vi "Main.vi"(11 "Module Admin":refnum<class "Delacor_lib_QMH_Cloneable Module Admin.lvclass">) -> ()   [LabVIEW 2024, in "Cloneable Subpanel.lvlib"]
doc: "This template is based off of the Queued Message Handler design pattern and the Queued Message Handler project template that ships with LabVIEW.\n\nThe main difference is that the queue is private to this module and communication between modules is performed via Broadcast and Request events.\n\nRequest events are wrapped in public API methods and are handled in the Event Handling Loop (EHL) of this VI. Any module can register for Broadcast events sent by this module. The EHL generates messages based on user interface actions.\n\nThe Message Handling Loop (MHL) processes messages generated by the EHL, or by other messages. The messages are string values, so new messages can be added easily to the Message Cases case structure in the MHL. Each message cluster can also provide an optional value for Message Data, which is a variant that can be converted to whatever message-specific data is required.\n_____\nBased on DQMH Dev Tools: Project Template 7.1.0.1499."
uses:
  Cloneable Subpanel.lvlib
  <vilib>/Delacor/Delacor QMH/Libraries/Message Queue_class/Delacor_lib_QMH_Message Queue.lvclass
  Module Data--cluster.ctl
  <vilib>/Utility/miscctls.llb/LVPointTypeDef.ctl
  <vilib>/Delacor/Delacor QMH/Libraries/Message Queue_class/Delacor_lib_QMH_Enqueue Message (Single).vi
  Stop Argument--cluster.ctl
  <vilib>/Delacor/Delacor QMH/Libraries/Cloneable Module Admin_class/Delacor_lib_QMH_Cloneable Module Admin.lvclass
  Draw FP in SubPanel Argument--cluster.ctl
  Remove from SubPanel Argument--cluster.ctl
panel:
  out "error out":errorcluster
  out "Status":string
  in  "Simulate EHL Error":bool
  in  "Simulate MHL Error":bool
  # "Other processes communicate with this Module via its Public API (wrappers for its Request Events).\n\nThis Module communicates with other processes via its Broadcast Events.\nAny process that wants to receive these messages can register for this module's Broadcast events."
  # "This template is for the DQMH framework. See the block diagram for more information on how to use this template."
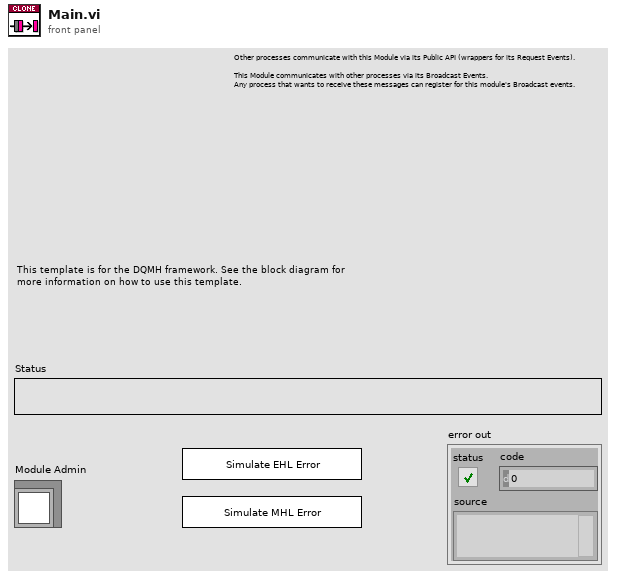
[diagram p1: front panel]
types:
  T1 = typedef "Cloneable Subpanel.lvlib/Request Events--cluster.ctl" = cluster{"Stop Module":refnum<user-event>, "Show Panel":refnum<user-event>, "Hide Panel":refnum<user-event>, "Show Diagram":refnum<user-event>, "Get Module Execution Status":refnum<user-event>, "Draw FP in SubPanel":refnum<user-event>, "Remove from SubPanel":refnum<user-event>}
  T2 = typedef "Cloneable Subpanel.lvlib/Module Data--cluster.ctl" = cluster{"Status":string, "Sub Panel":refnum<vi>}
  T3 = enum32{"invalid lock state", "Not Locked", "Locked (No Password)", "Password-protected"}
  T4 = typedef "Cloneable Subpanel.lvlib/Stop Argument--cluster.ctl" = cluster{"Module ID":i32, "Origin":string, "Exit via Stop Module Req?":bool, "Wait for Module to stop?":bool}
  T5 = typedef "Cloneable Subpanel.lvlib/Draw FP in SubPanel Argument--cluster.ctl" = cluster{"Module ID":i32, "Sub Panel":refnum<vi>}
  T6 = typedef "Cloneable Subpanel.lvlib/Remove from SubPanel Argument--cluster.ctl" = cluster{"Module ID":i32, "Boolean":bool}
  T7 = typedef "LVPointTypeDef.ctl" = cluster{"Horizontal":i16, "Vertical":i16}
  T8 = enum32{"Invalid", "Standard", "Closed", "Hidden", "Minimized", "Maximized"}
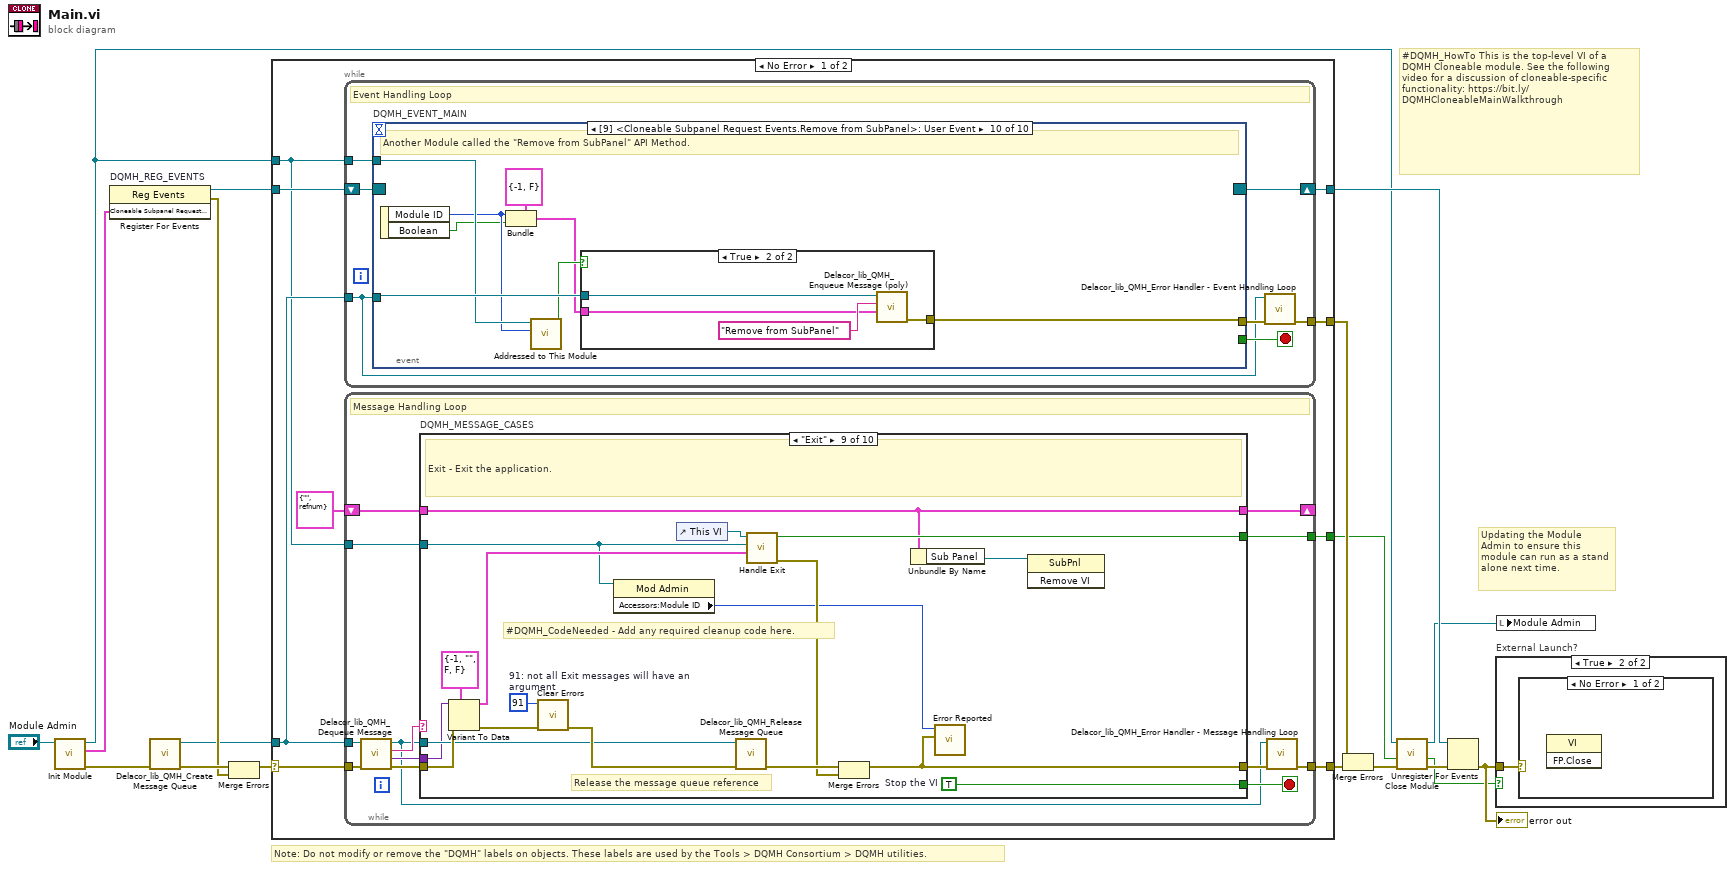
[diagram p0: block diagram]
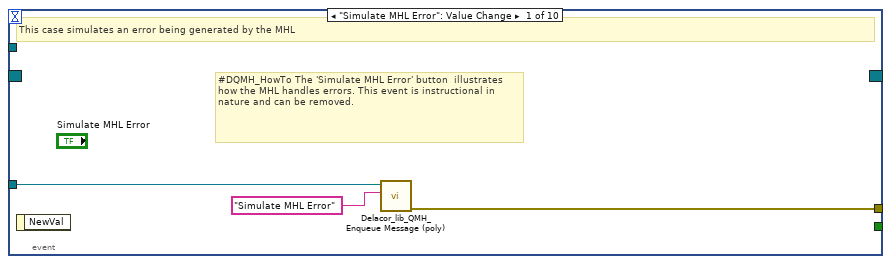
[diagram p2: hidden frame]
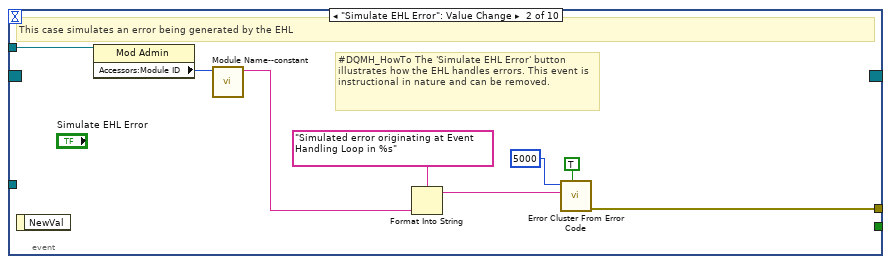
[diagram p3: hidden frame]
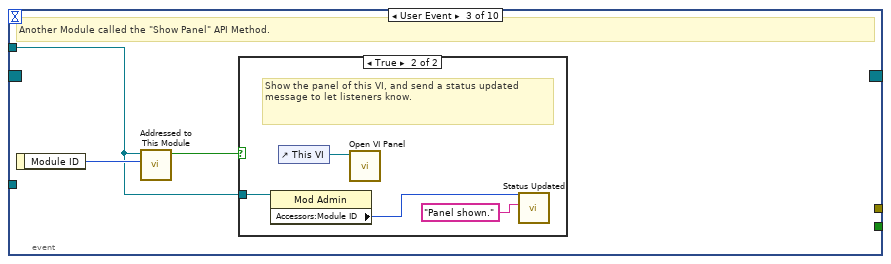
[diagram p4: hidden frame]
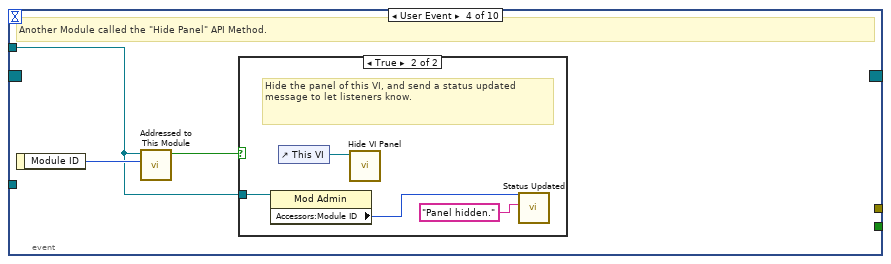
[diagram p6: hidden frame]
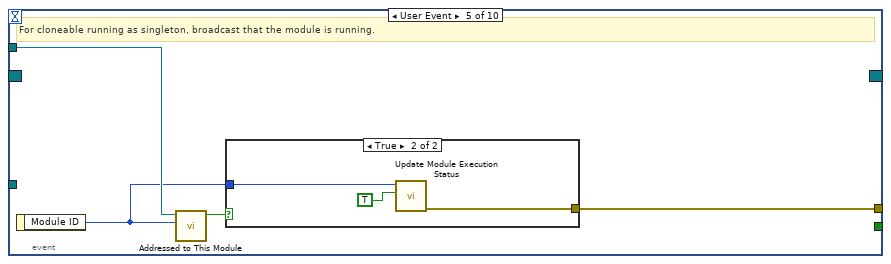
[diagram p8: hidden frame]
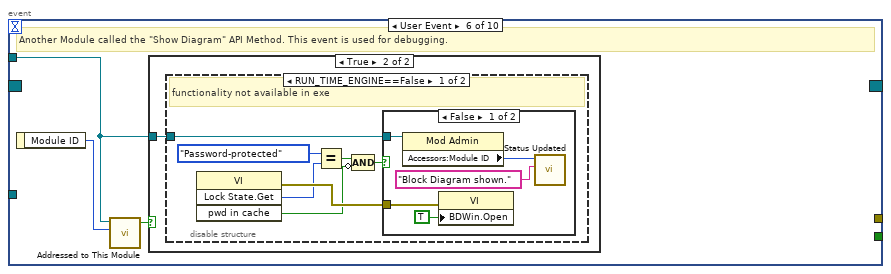
[diagram p10: hidden frame]
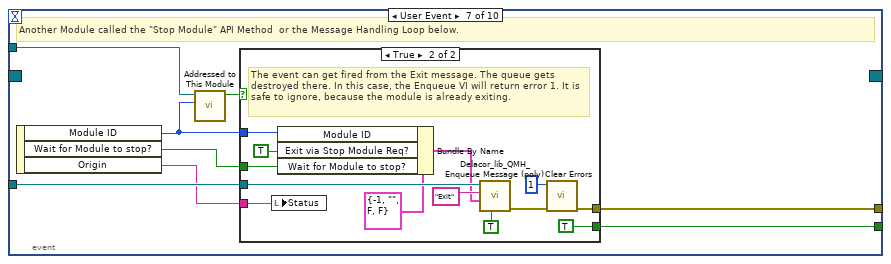
[diagram p14: hidden frame]
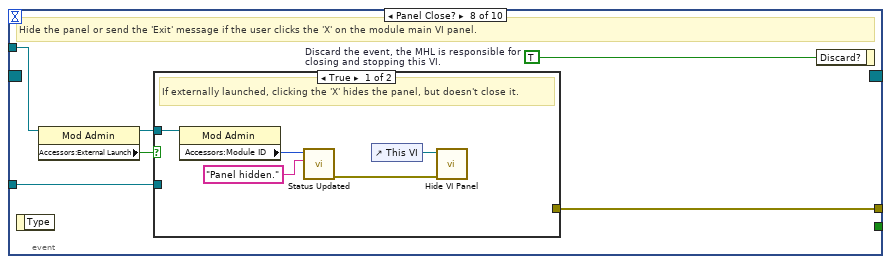
[diagram p16: hidden frame]
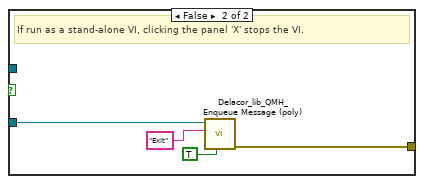
[diagram p17: hidden frame]
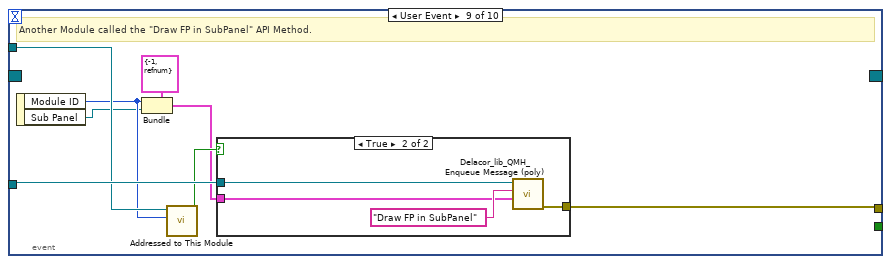
[diagram p18: hidden frame]
diagram:
  # "#DQMH_HowTo This is the top-level VI of a DQMH Cloneable module. See the following video for a discussion of cloneable-specific functionality: https://bit.ly/DQMHCloneableMainWalkthrough"
  # "Note: Do not modify or remove the \"DQMH\" labels on objects. These labels are used by the Tools > DQMH Consortium > DQMH utilities."
  # "Updating the Module Admin to ensure this module can run as a stand alone next time."
  n1 = call "Init Module.vi"("Cloneable Module Admin in"="Module Admin") -> ("error out"=w15:errorcluster, "Cloneable Subpanel Request Events"=w7:T1, "Cloneable Module Admin out"=w4:refnum<class "Delacor_lib_QMH_Cloneable Module Admin.lvclass">)  [unwired: 8 in]
  n2 = register-events "DQMH_REG_EVENTS"(w7) -> (reference out=w8:refnum<event-registration>, error out=w10:errorcluster)  [unwired: 2 in]
  n3 = call <vilib>:"Delacor_lib_QMH_Create Message Queue.vi"("error in"=w15) -> ("error out"=w12:errorcluster, "Message Queue"=w6:refnum<class "Delacor_lib_QMH_Message Queue.lvclass">)  [unwired: 9 in]
  n4 = Merge Errors(w12, w10) -> (w11:errorcluster)
  n5 = case shown="No Error" w11 {
    selector: w11 -> [w25 w287]
    tunnel: [w27 w286] -> w16
    tunnel: [w24 w285] -> w9
    tunnel: w8 -> [w22 w285]
    tunnel: w6 -> [w21 w278]
    tunnel: [w26 _] -> w17
    tunnel: w4 -> [w20 w281]
    tunnel: [w19 _] -> w2
    frame No Error {
      n6 = while {
        tunnel: w21 -> [w28]
        shift-right: [w31] -> w24
        shift-left: w22 -> [w32]
        tunnel: [w33] -> w26
        tunnel: w20 -> [w29]
        stop <- w30 stop-if-true
        # "Event Handling Loop"
        n7 = event "DQMH_EVENT_MAIN" shown="[9] <Cloneable Subpanel Request Events.Remove from SubPanel>: User Event" {
          selector: w32 -> [_ _ _ _ _ _ _ _ _ _]
          dyn-events: [_ _ _ _ _ _ _ _ _ _] -> w31
          timeout: _ -> [_ _ _ _ _ _ _ _ _ _]
          tunnel: [_ _ _ _ _ _ w86 _ _ _] -> w30
          tunnel: w28 -> [w36 _ _ _ _ _ w89 w106 w126 w138]
          tunnel: [w37 w45 _ _ w63 _ w90 w109 w119 w131] -> w34
          tunnel: w29 -> [_ w44 w46 w53 w61 w67 w88 w107 w124 w136]
          event "Simulate MHL Error": Value Change {
            # "#DQMH_HowTo The 'Simulate MHL Error' button  illustrates how the MHL handles errors. This event is instructional in nature and can be removed."
            # "This case simulates an error being generated by the MHL"
            n8 = event-data() -> ()  [unwired: 1 in, 1 out]
            n9 = call-poly <vilib>:"Delacor_lib_QMH_Enqueue Message (poly).vi"("Message"="Simulate MHL Error", "Message Queue in"=w36) -> ("error out"=w37:errorcluster)  [unwired: 8 in, 1 out]
          }
          event "Simulate EHL Error": Value Change {
            # "#DQMH_HowTo The 'Simulate EHL Error' button  illustrates how the EHL handles errors. This event is instructional in nature and can be removed."
            # "This case simulates an error being generated by the EHL"
            n10 = event-data() -> ()  [unwired: 1 in, 1 out]
            n11 = property on="Property Node" class="Mod Admin"(reference=w44) -> ("Accessors:Module ID"=w43:i32)  [unwired: 1 in, 2 out]
            n12 = call "Module Name--constant.vi"("Module ID"=w43) -> ("Module Name"=w38:string)  [unwired: 10 in]
            n13 = Format Into String(format string="Simulated error originating at Event Handling Loop in %s", w38) -> (resulting string=w41:string)  [unwired: 2 in, 1 out]
            n14 = call <vilib>:"Error Cluster From Error Code.vi"("show call chain? (False)"=TRUE, "error message (\"\")"=w41, "error code (0)"=5000) -> ("error out"=w45:errorcluster)  [unwired: 6 in]
          }
          event User Event {
            # "Another Module called the \"Show Panel\" API Method."
            n15 = event-data() -> ("Module ID"=w47:i32)  [unwired: 1 in]
            n16 = call "Addressed to This Module.vi"("Module ID from Argument"=w47, "Module Admin"=w46) -> ("Addressed to this instance?"=w48:bool)  [unwired: 8 in, 1 out]
            n17 = case shown="True" w48 {
              tunnel: w46 -> [_ w50]
              frame False {
              }
              frame True {
                # "Show the panel of this VI, and send a status updated message to let listeners know."
                n18 = property on="Property Node" class="Mod Admin"(reference=w50) -> ("Accessors:Module ID"=w49:i32)  [unwired: 1 in, 2 out]
                n19 = control-ref of="This VI"() -> (w52:refnum<vi>)
                n20 = call "Open VI Panel.vi"("VI"=w52) -> ()  [unwired: 10 in, 1 out]
                n21 = call "Status Updated.vi"("Status"="Panel shown." ("format string"), "Module ID"=w49) -> ()  [unwired: 9 in, 1 out]
              }
            }
          }
          event User Event {
            # "Another Module called the \"Hide Panel\" API Method."
            n22 = event-data() -> ("Module ID"=w54:i32)  [unwired: 1 in]
            n23 = call "Addressed to This Module.vi"("Module ID from Argument"=w54, "Module Admin"=w53) -> ("Addressed to this instance?"=w55:bool)  [unwired: 8 in, 1 out]
            n24 = case shown="True" w55 {
              tunnel: w53 -> [_ w57]
              frame False {
              }
              frame True {
                # "Hide the panel of this VI, and send a status updated message to let listeners know."
                n25 = property on="Property Node" class="Mod Admin"(reference=w57) -> ("Accessors:Module ID"=w56:i32)  [unwired: 1 in, 2 out]
                n26 = control-ref of="This VI"() -> (w59:refnum<vi>)
                n27 = call "Hide VI Panel.vi"("VI"=w59) -> ()  [unwired: 10 in, 1 out]
                n28 = call "Status Updated.vi"("Status"="Panel hidden." ("format string"), "Module ID"=w56) -> ()  [unwired: 9 in, 1 out]
              }
            }
          }
          event User Event {
            # "For cloneable running as singleton, broadcast that the module is running."
            n29 = event-data() -> ("Module ID"=w60:i32)  [unwired: 1 in]
            n30 = call "Addressed to This Module.vi"("Module ID from Argument"=w60, "Module Admin"=w61) -> ("Addressed to this instance?"=w62:bool)  [unwired: 8 in, 1 out]
            n31 = case shown="True" w62 {
              tunnel: [_ w66] -> w63
              tunnel: w60 -> [_ w65]
              frame False {
              }
              frame True {
                n32 = call "Update Module Execution Status.vi"("Running?"=TRUE, "Module ID"=w65) -> ("error out"=w66:errorcluster)  [unwired: 9 in]
              }
            }
          }
          event User Event {
            # "Another Module called the \"Show Diagram\" API Method. This event is used for debugging."
            n33 = event-data() -> ("Module ID"=w68:i32)  [unwired: 1 in]
            n34 = call "Addressed to This Module.vi"("Module ID from Argument"=w68, "Module Admin"=w67) -> ("Addressed to this instance?"=w69:bool)  [unwired: 8 in, 1 out]
            n35 = case shown="True" w69 {
              tunnel: w67 -> [_ w70]
              frame False {
              }
              frame True {
                n36 = disable-structure shown="RUN_TIME_ENGINE==False" {
                  disable-tunnel: w70 -> [w71 _]
                  frame condition #0 (active) {
                    # "functionality not available in exe"
                    n37 = invoke on="Invoke Node" class="VI" method="Lock State.Get"() -> (error out=w77:errorcluster, "Get Lock State"=w76:T3, "pwd in cache"=w73:bool)  [unwired: 4 in, 1 out]
                    n38 = Equal?(x=T3."Password-protected", y=w76) -> (x = y?=w74:bool)
                    n39 = Compound Arithmetic op=AND(w74, invert w73) -> (w72:bool)
                    n40 = case shown="False" w72 {
                      tunnel: w77 -> [w82 _]
                      tunnel: w71 -> [w79 _]
                      frame False {
                        n41 = property on="Property Node" class="Mod Admin"(reference=w79) -> ("Accessors:Module ID"=w78:i32)  [unwired: 1 in, 2 out]
                        n42 = property on="Property Node" class="VI"(error in=w82, "BDWin.Open"=TRUE ("Block Diagram Window:Open")) -> ()  [unwired: 1 in, 2 out]
                        n43 = call "Status Updated.vi"("Status"="Block Diagram shown." ("format string"), "Module ID"=w78) -> ()  [unwired: 9 in, 1 out]
                      }
                      frame True {
                        # "Password-protected VI, and the password is not in the cache. Do not show the diagram."
                      }
                    }
                  }
                  frame condition #1 {
                  }
                }
              }
            }
          }
          event User Event {
            # "Another Module called the \"Stop Module\" API Method  or the Message Handling Loop below."
            n44 = event-data() -> ("Module ID"=w84:i32, "Wait for Module to stop?"=w85:bool, "Origin"=w83:string)  [unwired: 1 in]
            n45 = call "Addressed to This Module.vi"("Module ID from Argument"=w84, "Module Admin"=w88) -> ("Addressed to this instance?"=w87:bool)  [unwired: 8 in, 1 out]
            n46 = case shown="True" w87 {
              tunnel: [_ w102] -> w90
              tunnel: w89 -> [_ w98]
              tunnel: [_ TRUE] -> w86
              tunnel: w85 -> [_ w93]
              tunnel: w84 -> [_ w95]
              tunnel: w83 -> [_ w91]
              frame False {
              }
              frame True {
                # "The event can get fired from the Exit message. The queue gets destroyed there. In this case, the Enqueue VI will return error 1. It is safe to ignore, because the module is already exiting."
                n47 = local write "Status"(w91) -> ()
                n48 = Bundle By Name(cluster=T4 {"Module ID"=-1, "Origin"="", "Exit via Stop Module Req?"=FALSE, "Wait for Module to stop?"=FALSE} ("Stop Argument"), "Module ID"=w95, "Exit via Stop Module Req?"=TRUE, "Wait for Module to stop?"=w93) -> (w92:T4)
                n49 = call-poly <vilib>:"Delacor_lib_QMH_Enqueue Message (poly).vi"("Priority Message? (F)"=TRUE, "Message Data"=w92, "Message"="Exit", "Message Queue in"=w98) -> ("error out"=w103:errorcluster)  [unwired: 6 in, 1 out]
                n50 = call <vilib>:"Clear Errors.vi"("error in (no error)"=w103, "specific error code to clear (0: all)"=1) -> ("error out"=w102:errorcluster)  [unwired: 4 in, 1 out]
              }
            }
          }
          event Panel Close? {
            w108 = TRUE  # Discard the event, the MHL is responsible for closing and stopping this VI.
            # "Hide the panel or send the 'Exit' message if the user clicks the 'X' on the module main VI panel."
            n51 = event-data() -> ()  [unwired: 1 in, 1 out]
            n52 = property on="Property Node" class="Mod Admin"(reference=w107) -> (reference out=w104:refnum<class "Delacor_lib_QMH_Cloneable Module Admin.lvclass">, "Accessors:External Launch"=w105:bool)  [unwired: 1 in, 1 out]
            n53 = case shown="True" w105 {
              tunnel: w106 -> [_ w117]
              tunnel: [_ w118] -> w109
              tunnel: w104 -> [w112 _]
              frame True {
                # "If externally launched, clicking the 'X' hides the panel, but doesn't close it."
                n54 = property on="Property Node" class="Mod Admin"(reference=w112) -> ("Accessors:Module ID"=w111:i32)  [unwired: 1 in, 2 out]
                n55 = call "Status Updated.vi"("Status"="Panel hidden." ("format string"), "Module ID"=w111) -> ("error out"=w110:errorcluster)  [unwired: 9 in]
                n56 = control-ref of="This VI"() -> (w114:refnum<vi>)
                n57 = call "Hide VI Panel.vi"("error in"=w110, "VI"=w114) -> ()  [unwired: 9 in, 1 out]
              }
              frame False {
                # "If run as a stand-alone VI, clicking the panel 'X' stops the VI."
                n58 = call-poly <vilib>:"Delacor_lib_QMH_Enqueue Message (poly).vi"("Priority Message? (F)"=TRUE, "Message"="Exit", "Message Queue in"=w117) -> ("error out"=w118:errorcluster)  [unwired: 7 in, 1 out]
              }
            }
            n59 = event-data ("Event Filter Node")("Discard?"=w108) -> ()  [unwired: 1 in, 1 out]
          }
          event User Event {
            # "Another Module called the \"Draw FP in SubPanel\" API Method."
            n60 = event-data() -> ("Module ID"=w121:i32, "Sub Panel"=w120:refnum<vi>)  [unwired: 1 in]
            n61 = Bundle(cluster=T5 {"Module ID"=-1, "Sub Panel"=refnum} ("Draw FP in SubPanel Argument"), "Module ID"=w121, "Sub Panel"=w120) -> (w122:T5)
            n62 = call "Addressed to This Module.vi"("Module ID from Argument"=w121, "Module Admin"=w124) -> ("Addressed to this instance?"=w125:bool)  [unwired: 8 in, 1 out]
            n63 = case shown="True" w125 {
              tunnel: w126 -> [_ w130]
              tunnel: w122 -> [_ w128]
              tunnel: [_ w127] -> w119
              frame False {
              }
              frame True {
                n64 = call-poly <vilib>:"Delacor_lib_QMH_Enqueue Message (poly).vi"("Message Data"=w128, "Message"="Draw FP in SubPanel", "Message Queue in"=w130) -> ("error out"=w127:errorcluster)  [unwired: 7 in, 1 out]
              }
            }
          }
          event User Event {
            # "Another Module called the \"Remove from SubPanel\" API Method."
            n65 = event-data() -> ("Module ID"=w133:i32, "Boolean"=w132:bool)  [unwired: 1 in]
            n66 = Bundle(cluster=T6 {"Module ID"=-1, "Boolean"=FALSE} ("Remove from SubPanel Argument"), "Module ID"=w133, "Boolean"=w132) -> (w134:T6)
            n67 = call "Addressed to This Module.vi"("Module ID from Argument"=w133, "Module Admin"=w136) -> ("Addressed to this instance?"=w137:bool)  [unwired: 8 in, 1 out]
            n68 = case shown="True" w137 {
              tunnel: w138 -> [_ w142]
              tunnel: w134 -> [_ w140]
              tunnel: [_ w139] -> w131
              frame False {
              }
              frame True {
                n69 = call-poly <vilib>:"Delacor_lib_QMH_Enqueue Message (poly).vi"("Message Data"=w140, "Message"="Remove from SubPanel", "Message Queue in"=w142) -> ("error out"=w139:errorcluster)  [unwired: 7 in, 1 out]
              }
            }
          }
        }
        n70 = call-dynamic "Delacor_lib_QMH_Error Handler - Event Handling Loop.vi"("error in"=w34, "Message Queue in"=w28) -> ("dup error in"=w33:errorcluster)  [unwired: 8 in, 1 out]
      }
      n71 = while {
        tunnel: w21 -> [w143]
        shift-right: [w150] -> _
        shift-left: T2 {"Status"="", "Sub Panel"=refnum} ("Data Cluster") -> [w151]
        tunnel: w25 -> [w154]
        tunnel: [w152] -> w27
        tunnel: w20 -> [w145]
        tunnel: [w144] -> w19
        stop <- w149 stop-if-true
        # "Message Handling Loop"
        n72 = call-dynamic "Delacor_lib_QMH_Dequeue Message.vi"("error in"=w154, "Message Queue in"=w143) -> ("error out"=w153:errorcluster, "Message Data"=w147:variant, "Message"=w148:string, "Message Queue out"=w146:refnum<class "Delacor_lib_QMH_Message Queue.lvclass">)  [unwired: 6 in]
        n73 = case "DQMH_MESSAGE_CASES" shown="\"Exit\"" w148 {
          selector: w148 -> [_ _ _ _ _ _ _ _ _ w267]
          tunnel: w146 -> [_ _ _ _ _ _ w221 _ w259 _]
          tunnel: w153 -> [w174 w178 w194 w209 w216 w218 w230 w247 w265 w276]
          tunnel: [w172 w178 w182 w199 w215 w218 w226 w246 w260 w277] -> w155
          tunnel: w151 -> [w165 w177 w193 w202 w214 w217 w225 w244 w249 w274]
          tunnel: [w164 w177 w180 w201 w214 w217 w225 w244 w249 w274] -> w150
          tunnel: [_ _ _ _ _ _ _ _ w258 _] -> w149
          tunnel: w147 -> [_ _ w191 w207 _ _ w224 _ w256 _]
          tunnel: w145 -> [w160 _ _ w197 _ _ w223 w242 w251 w273]
          tunnel: [_ _ _ _ _ _ _ _ w254 _] -> w144
          frame "Initialize" {
            w157 = "Initial Message" ("Initial Message")
            # "#DQMH_CodeNeeded - Initialize the appearance of the front panel."
            # "#DQMH_CodeNeeded - Initialize your state data here."
            # "Initialize - Any operation that needs to be done before the module can receive messages. Synchronize Caller Events.vi will inform Start Module.vi that the module has launched and is ready to receive messages. Module Did Init.vi will broadcast that the module initialized."
            n74 = call "Synchronize Caller Events.vi"("error in"=w174, "Module Admin"=w160) -> ("error out"=w173:errorcluster, "Module Admin out"=w159:refnum<class "Delacor_lib_QMH_Cloneable Module Admin.lvclass">)  [unwired: 8 in]
            n75 = property on="Property Node" class="Mod Admin"(reference=w159) -> ("Accessors:Module ID"=w156:i32, "Accessors:External Launch"=w161:bool)  [unwired: 1 in, 2 out]
            n76 = call "Module Name--constant.vi"("Module ID"=w156) -> ("Module Name"=w169:string)  [unwired: 10 in]
            n77 = property on="Property Node" class="VI"("Front Panel.Title"=w169) -> (reference out=w171:refnum<vi>, error out=w176:errorcluster)  [unwired: 2 in]
            n78 = Select(t=T8."Hidden" ("State"), s=w161, f=T8."Standard" ("State")) -> (s? t:f=w166:T8)
            n79 = invoke on="Invoke Node" class="VI" method="FP.Open"(reference=w171, error in=w176, "State"=w166) -> (reference out=w170:refnum<vi>, error out=w175:errorcluster)  [unwired: 2 in, 3 out]
            n80 = Bundle By Name(cluster=w165, "Status"=w157) -> (w164:T2)
            n81 = invoke on="Invoke Node" class="VI" method="FP.Center"(reference=w170, error in=w175) -> ()  [unwired: 1 in, 3 out]
            n82 = property on="Pane" class="Pane"("Origin"=T7 {"Horizontal"=0, "Vertical"=0}) -> ()  [unwired: 2 in, 2 out]
            n83 = call "Module Name--constant.vi"("Module ID"=w156) -> ("Module Name"=w162:string)  [unwired: 10 in]
            n84 = call "Module Did Init.vi"("error in"=w173, "Initialized?"=TRUE, "Origin"=w162, "Module ID"=w156) -> ("error out"=w172:errorcluster)  [unwired: 7 in]
            "Status" <- w157
          }
          frame "---Module Specific---" {
            # "Separator -- The following cases handle messages specific to this Module."
          }
          frame "Draw FP in SubPanel" {
            # "The VI Can't be inseted in a FP already Opened"
            # "Draw FP in SubPanel"
            n85 = Variant To Data(error in=w194, type=T5 {"Module ID"=-1, "Sub Panel"=refnum} ("Draw FP in SubPanel Argument"), Variant=w191) -> (data=w189:T5, error out=w192:errorcluster)
            n86 = Unbundle By Name(w189) -> ("Sub Panel"=w183:refnum<vi>)  [unwired: 1 out]
            n87 = control-ref of="This VI"() -> (w188:refnum<vi>)
            n88 = invoke class="VI" method="FP.Close"(reference=w188) -> (reference out=w187:refnum<vi>, error out=w186:errorcluster)  [unwired: 2 in, 1 out]
            n89 = call <vilib>:"Clear Errors.vi"("error in (no error)"=w186, "specific error code to clear (0: all)"=1149) -> ("error out"=w185:errorcluster)  [unwired: 4 in, 1 out]
            n90 = invoke class="SubPnl" method="Insert VI"(reference=w183, error in=w185, "VI Ref"=w187) -> (reference out=w179:refnum<vi>, error out=w181:errorcluster)  [unwired: 1 in, 2 out]
            n91 = Merge Errors(w192, w181) -> (w182:errorcluster)
            n92 = Bundle By Name(cluster=w193, "Sub Panel"=w179) -> (w180:T2)
          }
          frame "Remove from SubPanel" {
            # "Remove from SubPanel"
            n93 = Variant To Data(error in=w209, type=T6 {"Module ID"=-1, "Boolean"=FALSE} ("Remove from SubPanel Argument"), Variant=w207) -> (data=w205:T6, error out=w208:errorcluster)
            n94 = Unbundle By Name(w202) -> ("Sub Panel"=w204:refnum<vi>)
            n95 = property class="Mod Admin"(reference=w197) -> ("Accessors:Module ID"=w196:i32)  [unwired: 1 in, 2 out]
            n96 = Unbundle By Name(w205) -> ("Module ID"=w195:i32)  [unwired: 1 out]
            n97 = Not A Number/Path/Refnum?(number/path/refnum=w204) -> (NaN/Path/Refnum?=w203:bool)
            n98 = case shown="True" w203 {
              tunnel: w204 -> [w211 _]
              tunnel: [w210 _] -> w198
              tunnel: w196 -> [_ w212]
              tunnel: w195 -> [_ _]
              frame False {
                n99 = invoke class="SubPnl" method="Remove VI"(reference=w211) -> (error out=w210:errorcluster)  [unwired: 2 in, 2 out]
              }
              frame True {
                n100 = call "Status Updated.vi"("Status"="The Subpanel Ref is Nul, you must call 'Draw FP in Subpanel' Request First", "Module ID"=w212) -> ()  [unwired: 9 in, 1 out]
              }
            }
            n101 = Merge Errors(w208, w198) -> (w199:errorcluster)
            n102 = Bundle By Name(cluster=w202, "Sub Panel"=refnum<vi> refnum) -> (w201:T2)
          }
          frame "---Copy This Frame---" {
            # "Duplicate this frame when creating new messages.  Change this comment in the duplicated frame to describe this message."
            n103 = Merge Errors(w216) -> (w215:errorcluster)
          }
          frame "---Exit and Error Handling---" {
            # "Separator - the following cases handle errors and exit messages."
          }
          frame "Error" {
            # "#DQMH_CodeRecommended - If the module is running in standalone mode (External Launch = FALSE), this code will pop up an error dialog and call the 'Exit' message if an error occurs. Add more fine-grained error management here."
            # "Error - Check the error message data and respond accordingly. This message is sent by the \"Error Handler\" VIs at the end of each loop in this application."
            n104 = property on="Property Node" class="Mod Admin"(reference=w223) -> ("Accessors:External Launch"=w222:bool, "Accessors:Module ID"=w220:i32)  [unwired: 1 in, 2 out]
            n105 = Variant To Data(error in=w230, type=errorcluster {"status"=FALSE, "code"=0, "source"=""} ("error constant"), Variant=w224) -> (data=w219:errorcluster, error out=w228:errorcluster)
            n106 = local write "error out"(w219) -> ()
            n107 = call "Error Reported.vi"("Error"=w219, "Module ID"=w220) -> ()  [unwired: 9 in, 1 out]
            n108 = case shown="False" w222 {
              tunnel: [w235 _] -> w227
              tunnel: w221 -> [w233 _]
              tunnel: w219 -> [w234 _]
              frame False {
                n109 = disable-structure shown="Default" {
                  disable-tunnel: w234 -> [w236 _]
                  frame condition #0 (active) {
                    # "If the module is running standalone, then pop up an error dialog and call the \"Exit\" message."
                    n110 = call <vilib>:"Simple Error Handler.vi"("error in (no error)"=w236) -> ()  [unwired: 4 in, 5 out]
                  }
                  frame condition #1 {
                    # "To prevent the Simple Error Handler VI from being loaded (e.g. when deploying to a Real-Time target), add the Conditional Disable Symbol \"DQMH_Disable_SEH\" to your project and set it to TRUE."
                  }
                }
                n111 = call-poly <vilib>:"Delacor_lib_QMH_Enqueue Message (poly).vi"("Priority Message? (F)"=TRUE, "Message"="Exit", "Message Queue in"=w233) -> ("error out"=w235:errorcluster)  [unwired: 7 in, 1 out]
              }
              frame True {
                # "If the module was launched externally, calling the Error Reported broadcast VI is the only action performed by the \"Error\" message. The module's caller can then process the error appropriately."
              }
            }
            n112 = Merge Errors(w228, w227) -> (w226:errorcluster)
          }
          frame "Simulate MHL Error" {
            # "#DQMH_HowTo The 'Simulate MHL Error' button  illustrates how the MHL handles errors. This event is instructional in nature and can be removed."
            # "Simulate an error occurring at the MHL"
            n113 = property on="Property Node" class="Mod Admin"(reference=w242) -> ("Accessors:Module ID"=w243:i32)  [unwired: 1 in, 2 out]
            n114 = call "Module Name--constant.vi"("Module ID"=w243) -> ("Module Name"=w238:string)  [unwired: 10 in]
            n115 = Format Into String(format string="Simulated error originating at Message Handling Loop in %s", w238) -> (resulting string=w239:string)  [unwired: 2 in, 1 out]
            n116 = call <vilib>:"Error Cluster From Error Code.vi"("show call chain? (False)"=TRUE, "error message (\"\")"=w239, "error code (0)"=5001) -> ("error out"=w245:errorcluster)  [unwired: 6 in]
            n117 = Merge Errors(w247, w245) -> (w246:errorcluster)
          }
          frame "Exit" {
            w257 = 91  # 91: not all Exit messages will have an argument
            w258 = TRUE  # Stop the VI
            # "Release the message queue reference"
            # "#DQMH_CodeNeeded - Add any required cleanup code here."
            # "Exit - Exit the application."
            n118 = Variant To Data(error in=w265, type=T4 {"Module ID"=-1, "Origin"="", "Exit via Stop Module Req?"=FALSE, "Wait for Module to stop?"=FALSE} ("Stop Argument"), Variant=w256) -> (data=w253:T4, error out=w261:errorcluster)
            n119 = call <vilib>:"Clear Errors.vi"("error in (no error)"=w261, "specific error code to clear (0: all)"=w257) -> ("error out"=w264:errorcluster)  [unwired: 4 in, 1 out]
            n120 = property on="Property Node" class="Mod Admin"(reference=w251) -> ("Accessors:Module ID"=w250:i32)  [unwired: 1 in, 2 out]
            n121 = control-ref of="This VI"() -> (w252:refnum<vi>)
            n122 = call-dynamic "Delacor_lib_QMH_Release Message Queue.vi"("error in"=w264, "Message Queue"=w259) -> ("error out"=w263:errorcluster)  [unwired: 9 in]
            n123 = call "Handle Exit.vi"("Stop Argument"=w253, "Module Admin in"=w251, "VI reference"=w252) -> ("error out"=w262:errorcluster, "Wait for Stop?"=w254:bool)  [unwired: 7 in]
            n124 = Merge Errors(w263, w262) -> (w260:errorcluster)
            n125 = Unbundle By Name(w249) -> ("Sub Panel"=w248:refnum<vi>)
            n126 = call "Error Reported.vi"("Error"=w260, "Module ID"=w250) -> ()  [unwired: 9 in, 1 out]
            n127 = invoke class="SubPnl" method="Remove VI"(reference=w248) -> ()  [unwired: 2 in, 3 out]
          }
          frame Default {
            # "'Default' case only runs if there is a message that isn't defined in any of the other cases.  Output a programming error."
            n128 = property on="Property Node" class="Mod Admin"(reference=w273) -> ("Accessors:Module ID"=w272:i32)  [unwired: 1 in, 2 out]
            n129 = call "Module Name--constant.vi"("Module ID"=w272) -> ("Module Name"=w266:string)  [unwired: 10 in]
            n130 = Format Into String(format string="The invalid message string \"%s\" was received in the Message Handling Loop for module \"%s\".", w267, w266) -> (resulting string=w269:string)  [unwired: 2 in, 1 out]
            n131 = call <vilib>:"Error Cluster From Error Code.vi"("show call chain? (False)"=TRUE, "error message (\"\")"=w269, "error code (0)"=1) -> ("error out"=w275:errorcluster)  [unwired: 6 in]
            n132 = Merge Errors(w276, w275) -> (w277:errorcluster)
          }
        }
        n133 = call-dynamic "Delacor_lib_QMH_Error Handler - Message Handling Loop.vi"("error in"=w155, "Message Queue in"=w146) -> ("dup error in"=w152:errorcluster)  [unwired: 8 in, 1 out]
      }
    }
    frame Error {
      n134 = call "Synchronize Caller Events.vi"("Module Admin"=w281) -> ("Module Admin out"=w280:refnum<class "Delacor_lib_QMH_Cloneable Module Admin.lvclass">)  [unwired: 9 in, 1 out]
      n135 = property on="Property Node" class="Mod Admin"(reference=w280) -> ("Accessors:Module ID"=w279:i32)  [unwired: 1 in, 2 out]
      n136 = call-dynamic "Delacor_lib_QMH_Release Message Queue.vi"("error in"=w287, "Message Queue"=w278) -> ("error out"=w286:errorcluster)  [unwired: 9 in]
      n137 = call "Module Name--constant.vi"("Module ID"=w279) -> ("Module Name"=w284:string)  [unwired: 10 in]
      n138 = Format Into String(format string="An error occurred during initialization. %s is no longer running.", w284) -> (resulting string=w282:string)  [unwired: 2 in, 1 out]
      n139 = call "Error Reported.vi"("Additional Information"=w282, "Error"=w286, "Module ID"=w279) -> ()  [unwired: 8 in, 1 out]
    }
  }
  n140 = Merge Errors(w17, w16) -> (w18:errorcluster)
  n141 = call "Close Module.vi"("error in"=w18, "Wait for stop?"=w2, "Module Admin in"=w4) -> ("error out"=w14:errorcluster, "External Launch"=w1:bool, "Module Admin out"=w3:refnum<class "Delacor_lib_QMH_Cloneable Module Admin.lvclass">)  [unwired: 6 in]
  n142 = Unregister For Events(event registration refnum=w9, error in=w14) -> (error out=w13:errorcluster)
  "error out" <- w13
  n143 = case "External Launch?" shown="True" w1 {
    tunnel: w13 -> [_ w288]
    frame False {
    }
    frame True {
      n144 = case shown="No Error" w288 {
        frame No Error {
          n145 = invoke class="VI" method="FP.Close"() -> ()  [unwired: 3 in, 3 out]
        }
        frame Error {
          n146 = disable-structure shown="Default" {
            frame condition #0 (active) {
              n147 = invoke class="VI" method="FP.Open"("Activate"=TRUE ("Activate?")) -> ()  [unwired: 4 in, 5 out]
            }
            frame condition #1 {
              # "Don't show panel on error if running inside a built EXE."
            }
          }
        }
      }
    }
  }
  n148 = local write "Module Admin"(w3) -> ()
